vi "Extract Object Tokens.vi"(10 "JSON Object Descriptor":T1, 11 "attribute tokens":cluster{"token type":T4, T2}[](array[cluster])) -> (3 "Extracted Tokens":cluster{"token type":T4, T2}[](array[cluster]))   [LabVIEW 2020, in "Multi Error Cluster.lvlib"]
uses:
  <vilib>/MultiError/TokenizeJSON/Multi Error Cluster.lvlib
  <vilib>/MultiError/TokenizeJSON/JSON Token Values.ctl
  <vilib>/MultiError/Errors Cluster Multiple Errors/JSON Token Descriptor.ctl
  <vilib>/MultiError/TokenizeJSON/JSON Raw Token Values.ctl
  <vilib>/MultiError/Errors Cluster Multiple Errors/JSON Object Descriptor.ctl
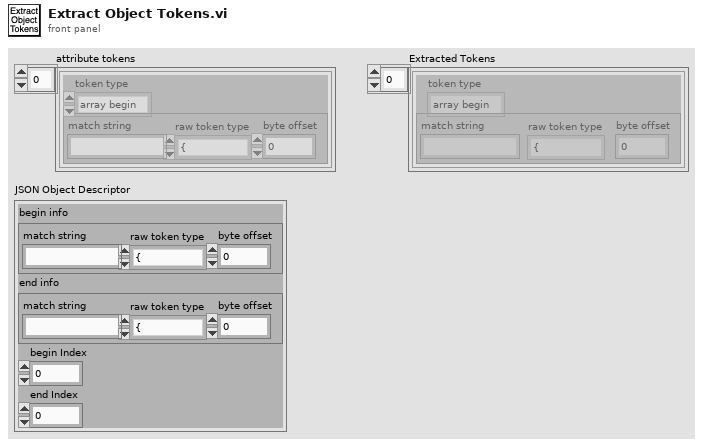
[diagram p1: front panel]
types:
  T1 = typedef "Multi Error Cluster.lvlib/JSON Object Descriptor.ctl" = cluster{"begin info":T2, "end info":T2, "begin Index":i32, "end Index":i32}
  T2 = typedef "Multi Error Cluster.lvlib/JSON Token Descriptor.ctl" = cluster{"match string":string, "raw token type":T3, "byte offset ":i32}
  T3 = typedef "Multi Error Cluster.lvlib/JSON Raw Token Values.ctl" = enum32{"{", "}", "[", "]", ",", ":", "\"", "number", "string", "true", "false", "null", "invalid"}
  T4 = typedef "Multi Error Cluster.lvlib/JSON Token Values.ctl" = enum32{"array begin", "array end", "object begin", "object end", "value", "invalid", "name"}
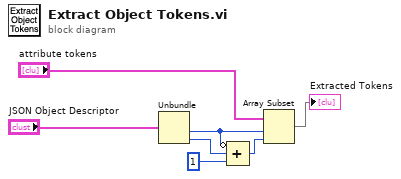
[diagram p0: block diagram]
diagram:
  n1 = Unbundle("JSON Object Descriptor") -> ("begin Index"=w4:i32, "end Index"=w2:i32)  [unwired: 2 out]
  n2 = Compound Arithmetic op=ADD(invert w4, w2, 1 ("value")) -> (w5:i32)
  n3 = Array Subset(array="attribute tokens", index=w4, length=w5) -> (→"Extracted Tokens":cluster{"token type":T4, T2}[])
